vi "raw_to_calibrated.vi"   [LabVIEW 2015, in "lv-calibration.lvlib"]
uses:
  lv-calibration.lvlib
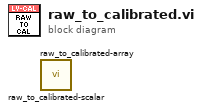
[diagram p0: block diagram]
diagram:
  n1 = call "raw_to_calibrated-scalar.vi"() -> ()  [unwired: 10 in, 2 out]
  n2 = call "raw_to_calibrated-array.vi"() -> ()  [unwired: 10 in, 2 out]
